vi "State Machine Template.vi"   [LabVIEW 2020, in "Publisher Subscriber.lvlib"]
uses:
  Publisher Subscriber.lvlib
  Controls/node refnum.ctl
  Controls/data cluster.ctl
  ae88ff53-e2b6-4b5a-85aa-5b466751ef77.vi
types:
  T1 = typedef "Publisher Subscriber.lvlib/node refnum.ctl" = refnum<k1>
  T2 = cluster{"Node Ref":T1, "E Ref":refnum<event-registration>, "Message":string, "Tout":i32}
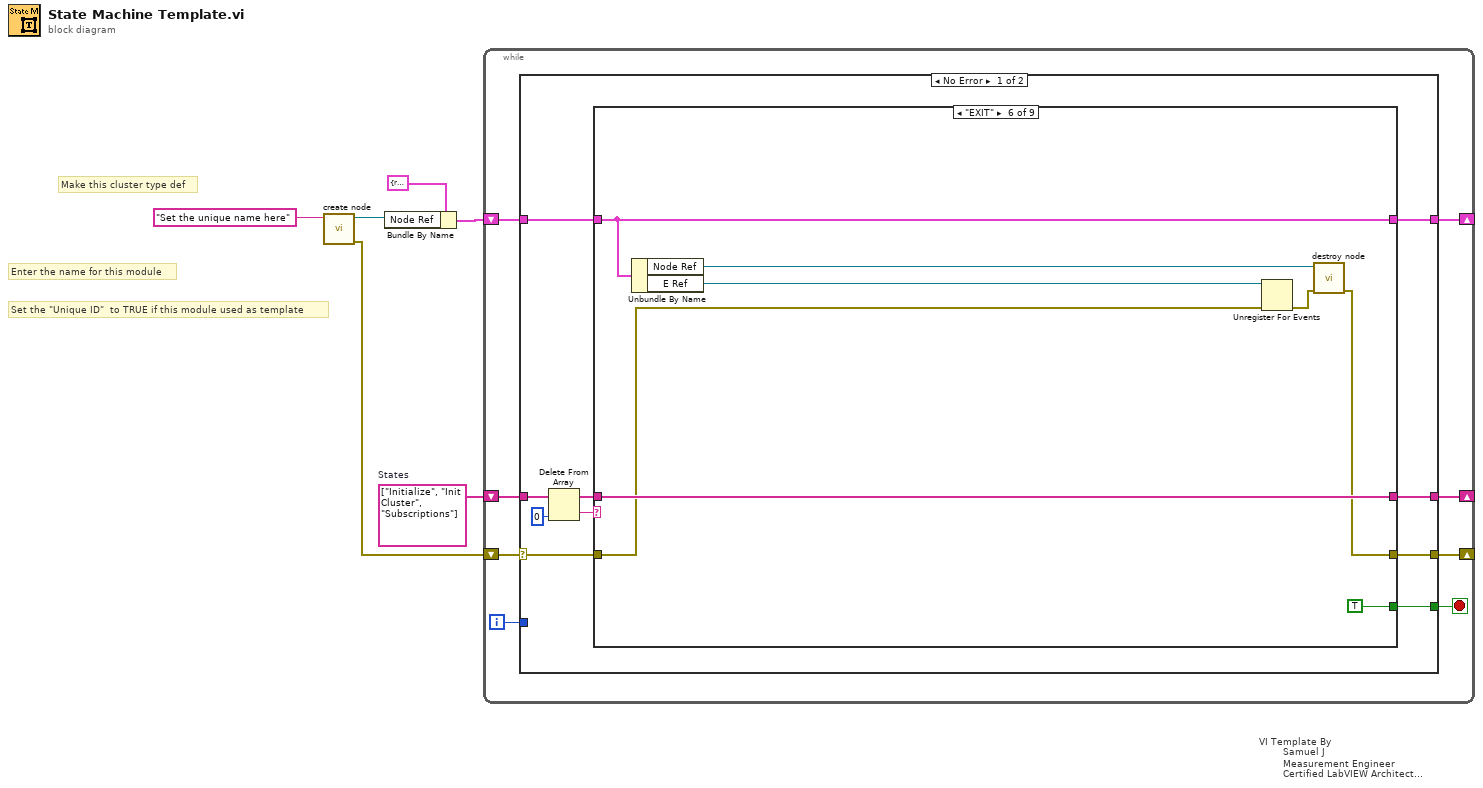
[diagram p0: block diagram]
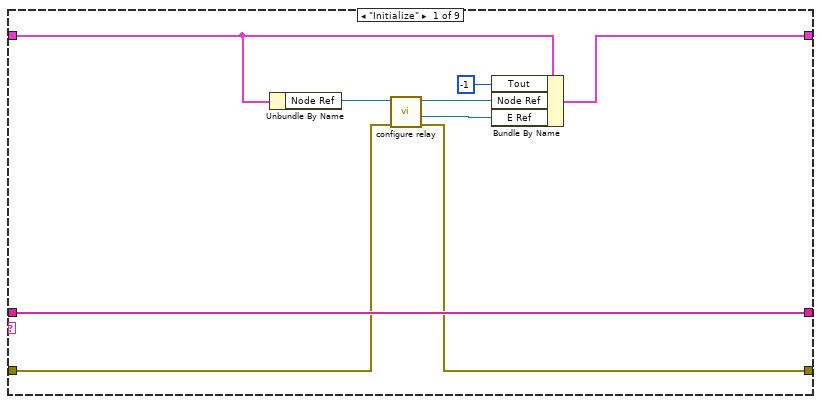
[diagram p2: hidden frame]
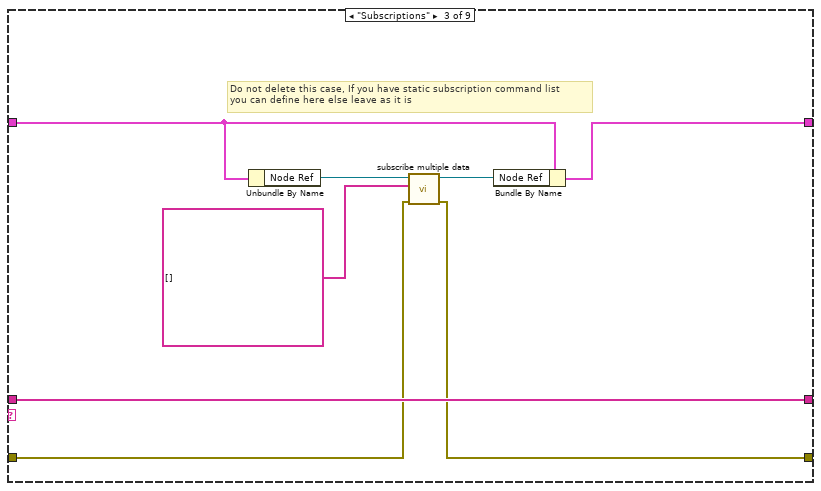
[diagram p4: hidden frame]
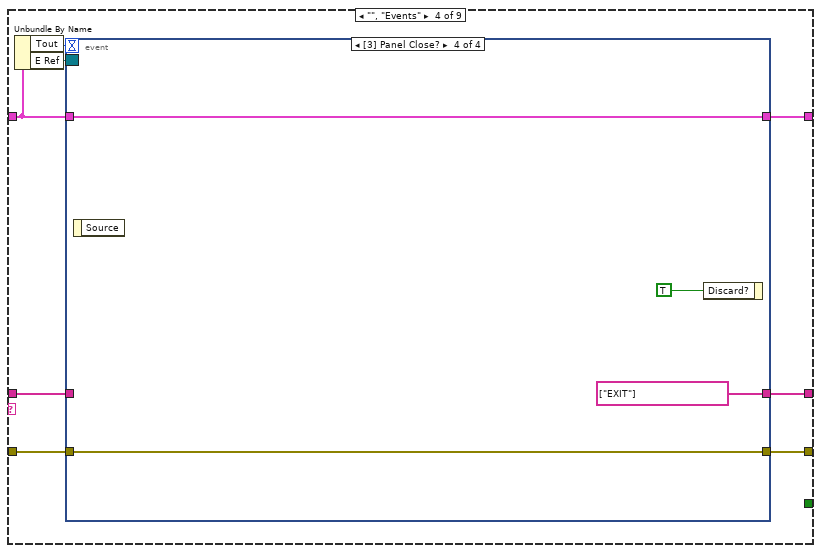
[diagram p5: hidden frame]
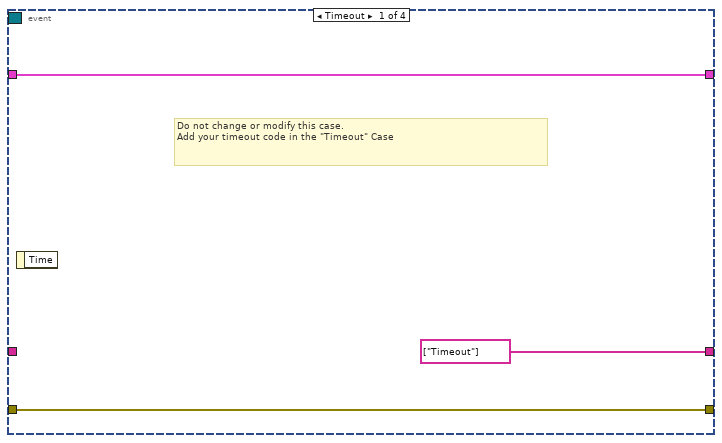
[diagram p6: hidden frame]
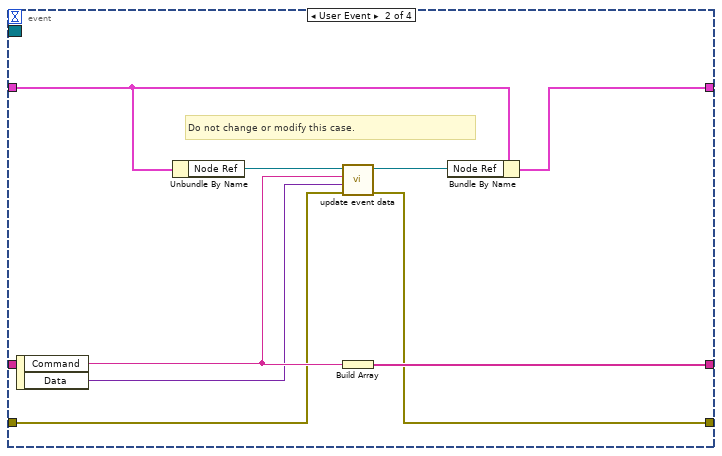
[diagram p7: hidden frame]
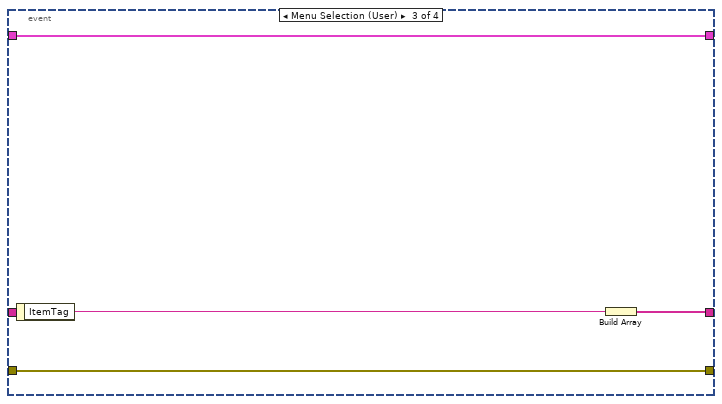
[diagram p8: hidden frame]
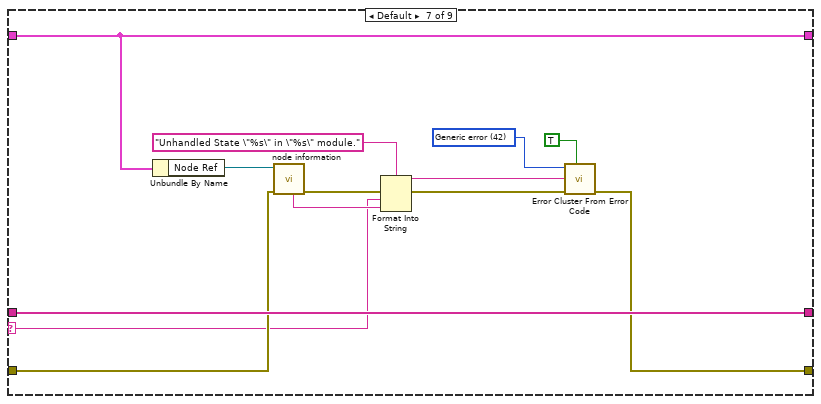
[diagram p10: hidden frame]
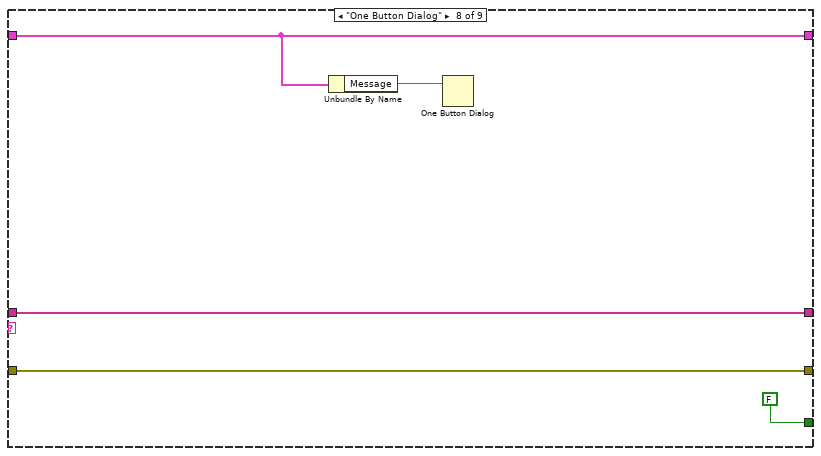
[diagram p11: hidden frame]
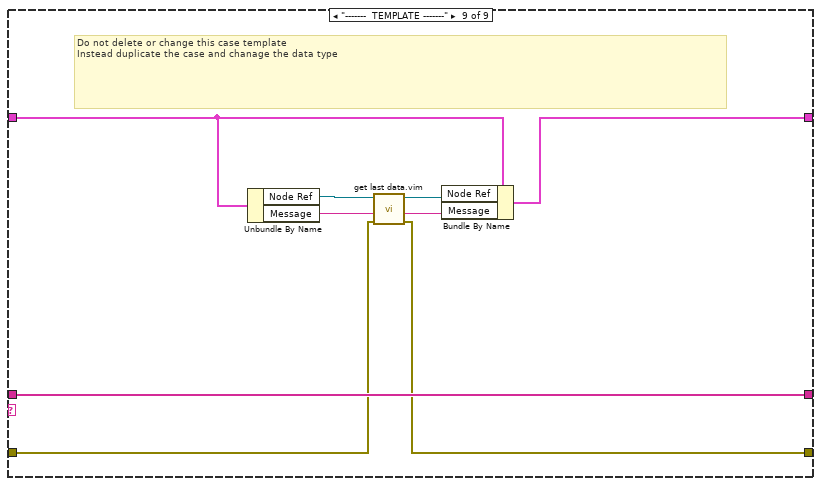
[diagram p12: hidden frame]
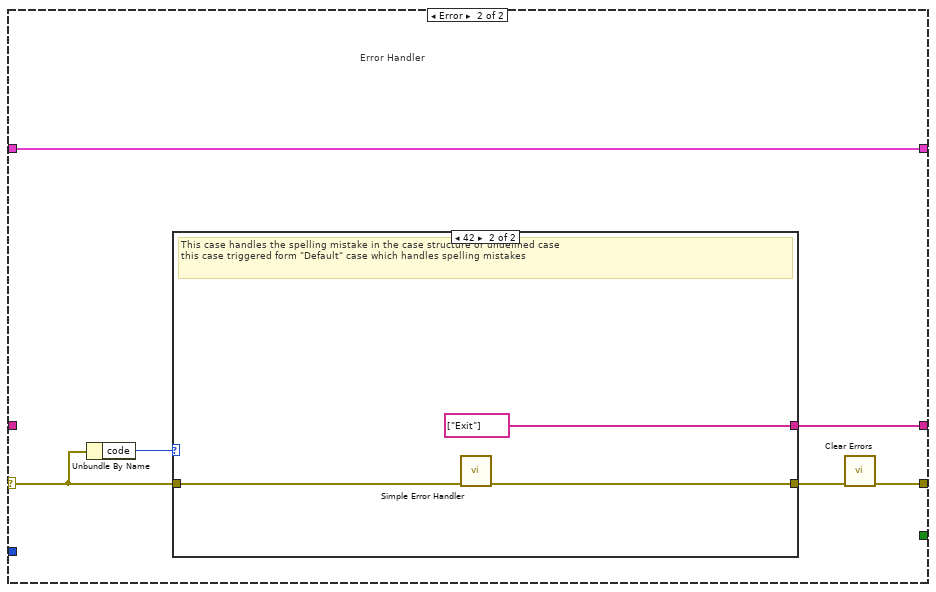
[diagram p13: hidden frame]
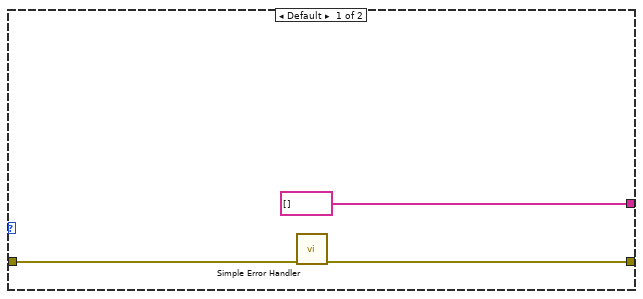
[diagram p14: hidden frame]
diagram:
  w6 = string[] ["Initialize", "Init Cluster", "Subscriptions"]  # States
  # "Set the \"Unique ID\"  to TRUE if this module used as template"
  # "Enter the name for this module"
  # "Make this cluster type def"
  n1 = call "create node.vi"("node name"="Set the unique name here" ("Subscriber name")) -> ("error out"=w1:errorcluster, "node ref out"=w3:T1)  [unwired: 9 in]
  n2 = Bundle By Name(cluster=T2 {"Node Ref"=refnum, "E Ref"=refnum, "Message"="", "Tout"=-1} ("Cluster"), "Node Ref"=w3) -> (w4:T2)
  n3 = while "VI Template By\n        Samuel J\n        Measurement Engineer\n        Certified LabVIEW Architect\n        Vestas Technology R&D Chennai" {
    shift-right: [w10] -> _
    shift-left: w6 -> [w14]
    shift-right: [w11] -> _
    shift-left: w1 -> [w13]
    shift-right: [w9] -> _
    shift-left: w4 -> [w12]
    i -> [w7]
    stop <- w8 stop-if-true
    n4 = case shown="No Error" w13 {
      selector: w13 -> [w19 w114]
      tunnel: w14 -> [w23 _]
      tunnel: w12 -> [w20 w116]
      tunnel: [w18 w112] -> w11
      tunnel: [w17 w111] -> w10
      tunnel: [w16 w116] -> w9
      tunnel: [w15 _] -> w8
      tunnel: w7 -> [_ _]
      frame No Error {
        n5 = Delete From Array(array=w23, index=0) -> (deleted portion=w22:string, array with subset deleted=w21:string[])  [unwired: 1 in]
        n6 = case shown="\"EXIT\"" w22 {
          selector: w22 -> [_ _ _ _ _ _ w84 _ _]
          tunnel: w21 -> [w33 w35 w44 w48 w74 w83 w96 w99 w110]
          tunnel: w20 -> [w30 w34 w41 w47 w73 w80 w87 w98 w107]
          tunnel: w19 -> [w27 w36 w38 w52 w75 w76 w86 w100 w104]
          tunnel: [w28 w36 w39 w50 w75 w79 w85 w100 w105] -> w18
          tunnel: [w33 w35 w44 w49 w74 w83 w96 w99 w110] -> w17
          tunnel: [w31 w34 w42 w51 w73 w80 w87 w98 w108] -> w16
          tunnel: [_ _ _ _ _ TRUE ("Exit") _ FALSE ("Exit") _] -> w15
          frame "Initialize" {
            n7 = Unbundle By Name(w30) -> ("Node Ref"=w32:T1)
            n8 = call "configure relay.vi"("error in"=w27, "Node Ref in"=w32) -> ("error out"=w28:errorcluster, "Event Reg Ref"=w25:refnum<event-registration>, "Node Ref out"=w29:T1)  [unwired: 7 in]
            n9 = Bundle By Name(cluster=w30, "Tout"=-1, "Node Ref"=w29, "E Ref"=w25) -> (w31:T2)
          }
          frame "Init Cluster" {
          }
          frame "Subscriptions" {
            # "Do not delete this case, If you have static subscription command list \nyou can define here else leave as it is"
            n10 = Unbundle By Name(w41) -> ("Node Ref"=w43:T1)
            n11 = call "subscribe multiple data.vi"("error in"=w38, "subriscription list[]"=string[] [], "refnum in"=w43) -> ("error out"=w39:errorcluster, "refnum out"=w40:T1)  [unwired: 7 in]
            n12 = Bundle By Name(cluster=w41, "Node Ref"=w40) -> (w42:T2)
          }
          frame "", "Events" {
            n13 = Unbundle By Name(w47) -> ("Tout"=w45:i32, "E Ref"=w46:refnum<event-registration>)
            n14 = event shown="[3] Panel Close?" {
              selector: w46 -> [_ _ _ _]
              dyn-events: _ -> [_ _ _ _]
              timeout: w45 -> [_ _ _ _]
              tunnel: w47 -> [w55 w57 w68 w71]
              tunnel: w52 -> [w54 w59 w65 w70]
              tunnel: [w55 w58 w68 w71] -> w51
              tunnel: [w54 w60 w65 w70] -> w50
              tunnel: [string[] ["Timeout"] ("States") w64 w66 string[] ["EXIT"] ("States")] -> w49
              tunnel: w48 -> [_ _ _ _]
              event Timeout {
                # "Do not change or modify this case. \nAdd your timeout code in the \"Timeout\" Case"
                n15 = event-data() -> ()  [unwired: 2 out]
              }
              event User Event {
                # "Do not change or modify this case."
                n16 = event-data() -> ("Command"=w62:string, "Data"=w61:variant)  [unwired: 1 out]
                n17 = Unbundle By Name(w57) -> ("Node Ref"=w63:T1)
                n18 = call "update event data.vi"("error in"=w59, "data type"=w61, "Command"=w62, "refnum in"=w63) -> ("error out"=w60:errorcluster, "refnum in"=w56:T1)  [unwired: 6 in]
                n19 = Build Array(w62) -> (w64:string[])
                n20 = Bundle By Name(cluster=w57, "Node Ref"=w56) -> (w58:T2)
              }
              event Menu Selection (User) {
                n21 = event-data() -> ("ItemTag"=w67:string)  [unwired: 1 out]
                n22 = Build Array(w67) -> (w66:string[])
              }
              event Panel Close? {
                n23 = event-data() -> ()  [unwired: 2 out]
                n24 = event-data("Discard?"=TRUE) -> ()  [unwired: 1 in, 1 out]
              }
            }
          }
          frame "Timeout" {
            # "Do not delete this case. Add your timeout code here else leave as it is."
          }
          frame "EXIT" {
            n25 = Unbundle By Name(w80) -> ("Node Ref"=w81:T1, "E Ref"=w78:refnum<event-registration>)
            n26 = Unregister For Events(event registration refnum=w78, error in=w76) -> (error out=w77:errorcluster)
            n27 = call "destroy node.vi"("error in"=w77, "refnum in"=w81) -> ("error out"=w79:errorcluster)  [unwired: 8 in, 1 out]
          }
          frame Default {
            w92 = 42 items=["No error", "Argument error", "Memory is full", "Out of zone", "End of file", "File already open", "Generic file I/O error", "File not found", "File permission error", "Disk is full", "Duplicate path", "Too many files open", "System feature not enabled", "Resource file not found", "Cannot add resource", "Resource not found", "Image not found", "Image memory error", "Pen does not exist", "Config type invalid", "Config token not found", "Config parse error", "Config memory error", "Bad external code format", "Bad external code offset", "External code not present", "Null window", "Destroy window error", "Null menu", "Print aborted", "Bad print record", "Print driver error", "Windows error during printing", "Memory error during printing", "Print dialog error", "Generic print error", "Invalid device refnum", "Device not found", "Device parameter error", "Device unit error", "Cannot open device", "Device call aborted", "Generic error", "Cancelled by user", "Object ID too low", "Object ID too high", "Object not in heap", "Unknown heap", "Unknown object (invalid DefProc)", "Unknown object (DefProc not in table)", "Message out of range", "Invalid (null) method", "Unknown message", "Manager call not supported", "Bad address", "Network operation in progress", "Network operation timed out", "Connection is busy", "Network attribute not supported", "Network error", "Address in use", "System out of memory", "Connection aborted", "Connection refused", "Not connected", "Already connected", "Connection closed", "Initialization error (interapplication manager)", "Bad occurrence", "Wait on unbound occurrence handler", "Occurrence queue overflow", "Datalog type conflict", "Unused", "Unrecognized type (interapplication manager)", "Memory corrupt", "Failed to make temporary DLL", "Old CIN version", "Drag socket not found", "Failed to load drop-object", "Failed to register OLE object", "Failed to release OLE object", "Format specifier type mismatch", "Unknown format specifier", "Too few format specifiers", "Too many format specifiers", "Scan failed", "Newer CIN version", "Error converting to variant", "Runtime menu error", "Password tampered", "Variant attribute not found", "Incompatible variant data type", "Event data is not available", "Event Store is not present", "Occurrence is not found", "Event Queue is not created", "Event info is not available", "Refnum passed is NULL", "Error retrieving Class GUID", "Error retrieving CoClass GUID", "Error retrieving TypeLib GUID.", "Bad built application magic bytes.", "Specific driver is different from the specific driver associated with the Logical Name.", "There is no session opened to the class driver.", "Max Error", "MAX - Error with config objects", "MAX - Error loading configuration", "MAX - Group not supported"]
            n28 = Unbundle By Name(w87) -> ("Node Ref"=w90:T1)
            n29 = call "node information.vi"("error in"=w86, "refnum in"=w90) -> ("error out"=w88:errorcluster, "this node name"=w89:string)  [unwired: 4 in, 4 out]
            n30 = Format Into String(format string="Unhandled State \"%s\" in \"%s\" module." ("message"), error in=w88, w84, w89) -> (resulting string=w93:string, error out=w94:errorcluster)  [unwired: 1 in]
            n31 = call <vilib>:"Error Cluster From Error Code.vi"("show call chain? (False)"=TRUE, "error in (no error)"=w94, "error message (\"\")"=w93, "error code (0)"=w92) -> ("error out"=w85:errorcluster)  [unwired: 5 out]
          }
          frame "One Button Dialog" {
            n32 = Unbundle By Name(w98) -> ("Message"=w101:string)
            n33 = One Button Dialog(message=w101) -> ()  [unwired: 2 out]
          }
          frame "-------  TEMPLATE -------" {
            # "Do not delete or change this case template \nInstead duplicate the case and chanage the data type"
            n34 = Unbundle By Name(w107) -> ("Node Ref"=w109:T1, "Message"=w103:string)
            n35 = call "get last data.vim"("error in"=w104, "data type"=w103, "refnum in"=w109) -> ("error out"=w105:errorcluster, "data out"=w102:string, "refnum out"=w106:T1)  [unwired: 5 in, 1 out]
            n36 = Bundle By Name(cluster=w107, "Node Ref"=w106, "Message"=w102) -> (w108:T2)
          }
        }
      }
      frame Error {
        # "Error Handler"
        n37 = Unbundle By Name(w114) -> ("code"=w115:i32)
        n38 = case shown="42" w115 {
          tunnel: w114 -> [w119 w122]
          tunnel: [w118 w121] -> w113
          tunnel: [string[] [] ("States") string[] ["Exit"] ("States")] -> w111
          frame Default {
            n39 = call <vilib>:"Simple Error Handler.vi"("error in (no error)"=w119) -> ("error out"=w118:errorcluster)  [unwired: 1 in, 7 out]
          }
          frame 42 {
            # "This case handles the spelling mistake in the case structure or undefined case\nthis case triggered form \"Default\" case which handles spelling mistakes"
            n40 = call <vilib>:"Simple Error Handler.vi"("error in (no error)"=w122) -> ("error out"=w121:errorcluster)  [unwired: 1 in, 7 out]
          }
        }
        n41 = call <vilib>:"Clear Errors.vi"("error in (no error)"=w113) -> ("error out"=w112:errorcluster)  [unwired: 1 in, 5 out]
      }
    }
  }
